vi "SENS_CORR_CSET_ACT.vi"(0 "VISA IN":refnum<visa-resource-name>, 1 "Calset":string, 2 "Apply Calset?":bool, 5 "error in":errorcluster, 7 "Channel":i32) -> (14 "VISA Out":refnum<visa-resource-name>, 19 "error out":errorcluster)   [LabVIEW 2018, in "PNA-X.lvlib"]
doc: "SENSe<cnum>:CORRection:CSET:ACTivate <string>, <bool> \nThis command replaces SENS:CORR:CSET:GUID \n(Read-Write) Selects and applies a Cal Set to the specified channel. \nUse SENS:CORR:CSET:CAT? to list the Cal Sets. \nParameters \n<cnum> Any existing channel number. If unspecified, value is set to 1 \n<string> Cal Set to make active. Specify the Cal Set by GUID or Name. Use \nSENS:CORR:CSET:CAT? to list the available Cal Sets in either format. \n<bool> Should the Cal Set stimulus values be applied to the channel. Choose from: \nON (1) Apply the Cal Set stimulus values to the channel. \nOFF (0) Do NOT apply the Cal Set stimulus values. If the Cal Set stimulus \nvalues do not match the channel stimulus values, then the following will occur: \n1689\n\nIf interpolation is ON, then interpolation will be attempted. This may fail if the \nchannel frequency is outside the range of the Cal Set. \nIf interpolation is OFF, the selection will be abandoned and an error is returned: \nExamples SENS:CORR:CSET:ACT \"My2Port\",1 \nsense:correction:cset:activate? name \n'returns \n\"My2Port\" \nQuery Syntax SENSe<cnum>:CORRection:CSET:ACTivate? [GUID|NAME] \nReturns the name of the Cal Set that is applied to the specified channel. Choose \nfrom GUID or NAME to specify which string is returned. If unspecified, the \nGUID of the Cal Set is returned. If no Cal Set is applied to the specified \nchannel, then \"No Calset Selected\" is returned. \nReturn Type String \nDefault Not Applicable \nSENSe:CORRection:CSET:CATalog? [char] \n(Read-only) Returns a list of Cal Sets. \nParameters \n<char> Optional argument. The list is returned in one of the following formats. Both \nreturn comma-separated string lists. \nGUID Cal Sets are listed by GUID (Default if unspecified). \nNAME Cal Sets are listed by Name \nExamples SENS:CORR:CSET:CAT? \n'Returns: \n{FD6F863E-9719-11d5-8D6C-00108334AE96},{1B03B2CE-971A-11d5-8D6C- \n00108334AE96} \nsense2:correction:cset:catalog? name \nDefault Not Applicable"
uses:
  PNA-X.lvlib
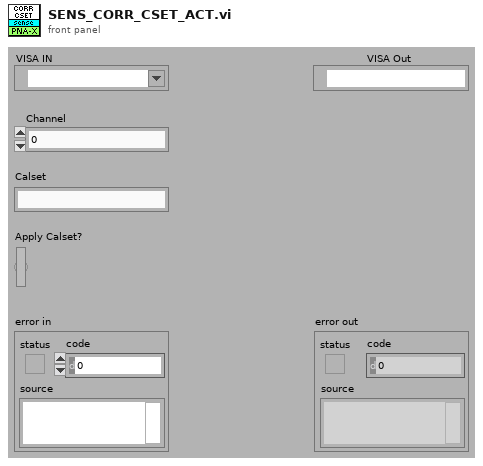
[diagram p1: front panel]
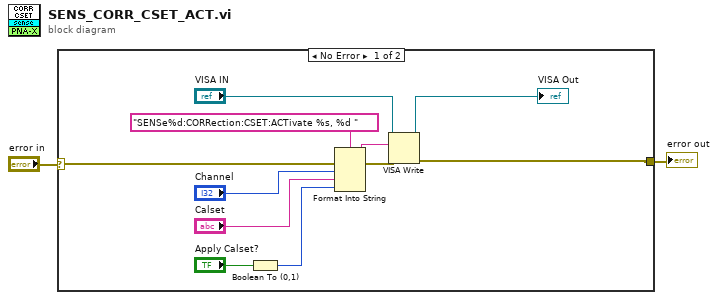
[diagram p0: block diagram]
diagram:
  n1 = case shown="No Error" "error in" {
    selector: "error in" -> [w13 w14]
    tunnel: [w8 w14] -> w1
    frame No Error {
      n2 = Boolean To (0,1)(Boolean="Apply Calset?") -> (0, 1=w3:i16)
      n3 = Format Into String(format string="SENSe%d:CORRection:CSET:ACTivate %s, %d " ("Cmdline"), error in=w13, "Channel", "Calset", w3) -> (resulting string=w11:string, error out=w12:errorcluster)  [unwired: 1 in]
      n4 = VISA Write(VISA resource name="VISA IN", write buffer=w11, error in (no error)=w12) -> (VISA resource name out=→"VISA Out":refnum<visa-resource-name>, error out=w8:errorcluster)  [unwired: 1 out]
    }
    frame Error {
    }
  }
  "error out" <- w1
